vi "MeasLeakRate11.vi"() -> ()   [LabVIEW 2011]
panel:
  out "fit":cluster{"element":dbl, "Value":dbl}[](array[cluster])
  out "T-T0,P":cluster{"element":dbl, "element":dbl}[](array[cluster])
  out "t0":dbl format="%#_8f"
  out "XY Graph":T1(graph)
  out "S00":i32
  out "S20":dbl
  out "S11":dbl
  out "S10":dbl
  out "S01":dbl
  out "T,P":cluster{"element":dbl, "element":dbl}[](array[cluster])
  out "dPdt":dbl
  out "P0":dbl
  out "average P (Torr)":string
  in  "Control Valve local":bool
  in  "Exhaust Local":bool
  in  "Exhaust Close":bool
  in  "Exhaust Open":bool
  in  "Control Close":bool
  in  "Control Open":bool
  in  "reset":bool
  in  "# points to watch":i32=60
  out "leak rate (Torr/min)":string
  out "P":dbl
  out "first":bool=TRUE
  in  "interval (s)":dbl=0.5
  in  "stop":bool
  out "P(Torr)":string
  # "Pressure control valve:"
  # "Exahaust valve:"
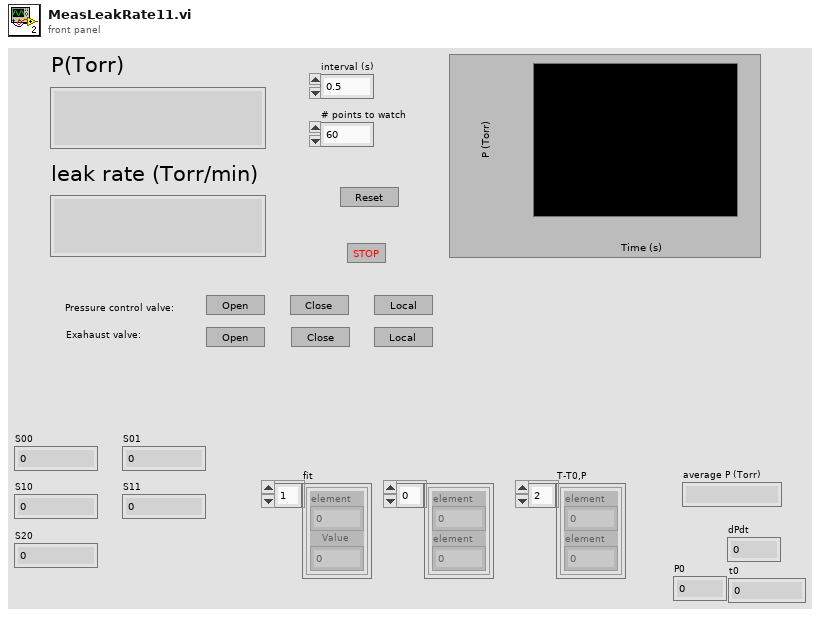
[diagram p1: front panel]
types:
  T1 = cluster{"Value":cluster{"element":dbl, "element":dbl}[]}[]
  T2 = cluster{"Value":cluster{"element":dbl, "Value":dbl}[]}[]
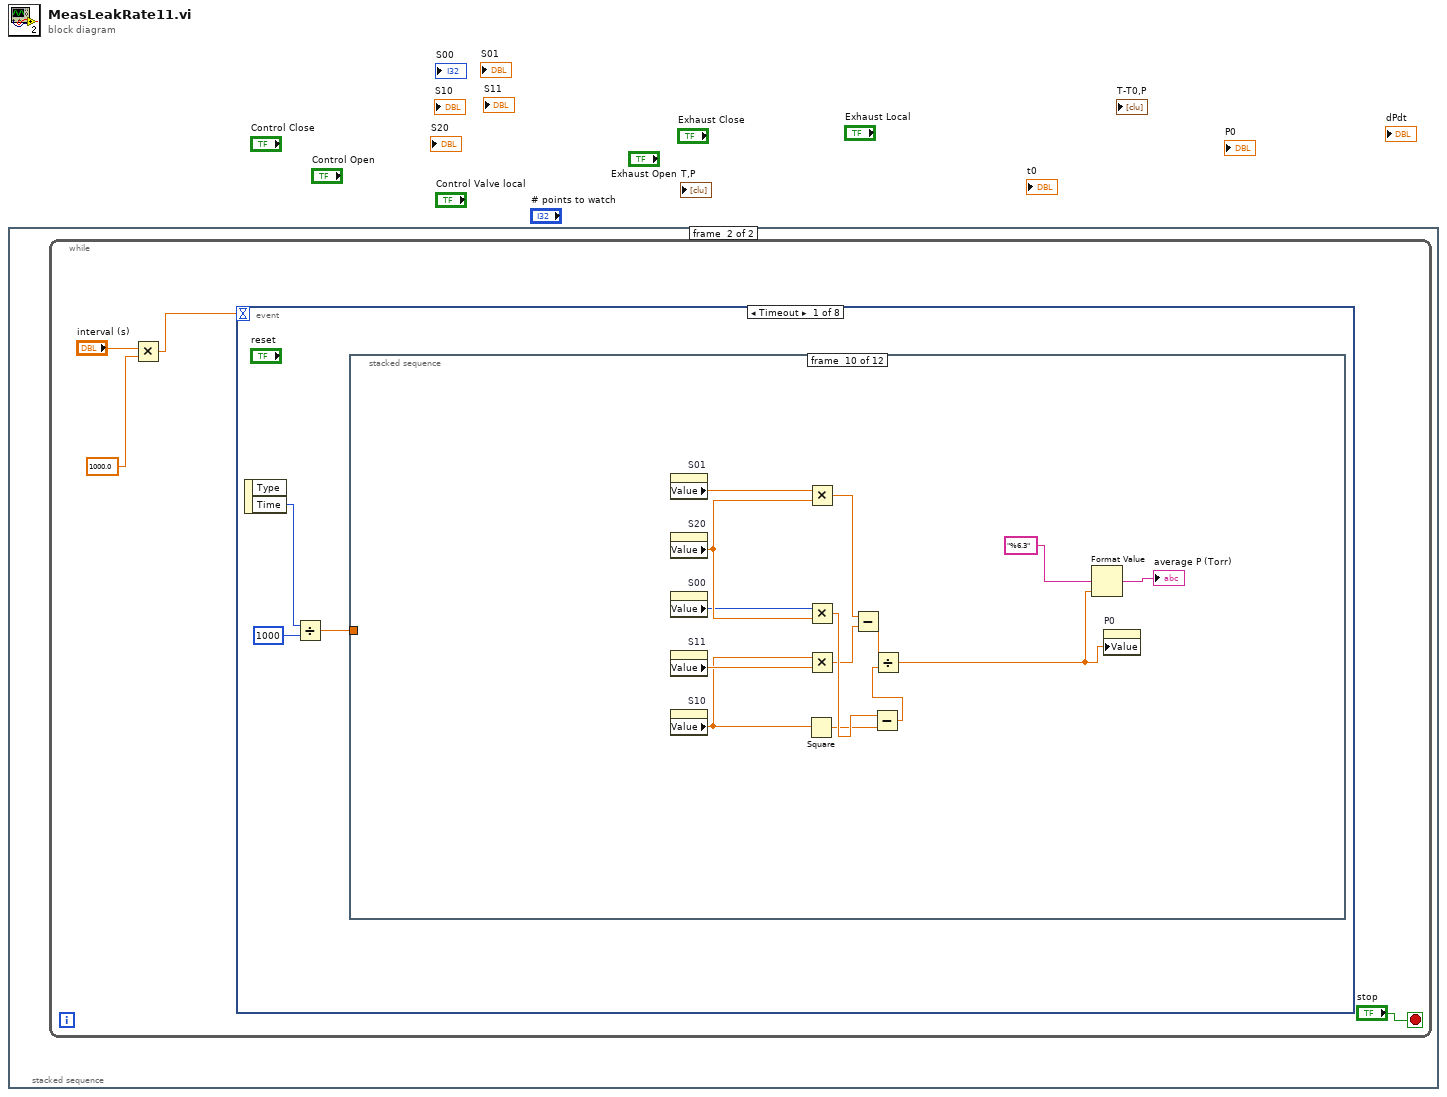
[diagram p0: block diagram]
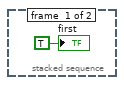
[diagram p2: hidden frame]
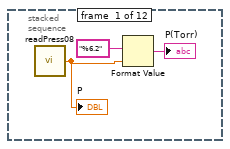
[diagram p3: hidden frame]
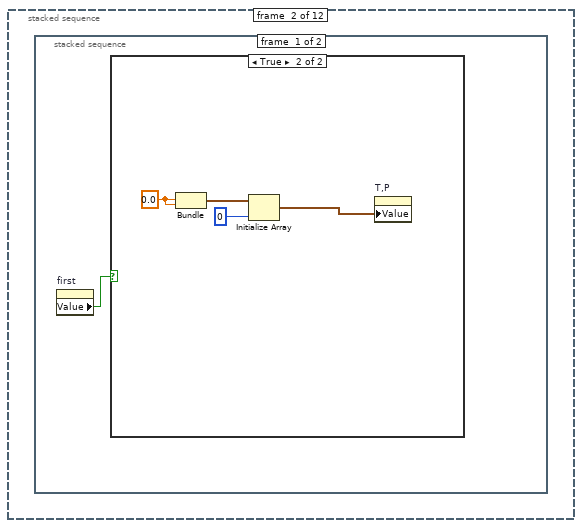
[diagram p4: hidden frame]
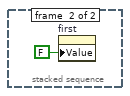
[diagram p6: hidden frame]
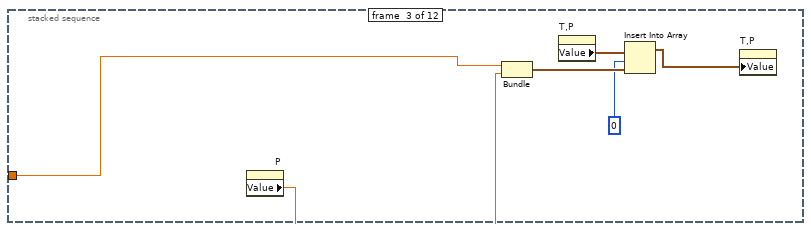
[diagram p7: hidden frame]
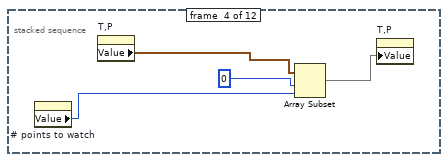
[diagram p8: hidden frame]
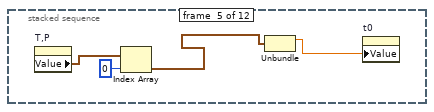
[diagram p9: hidden frame]
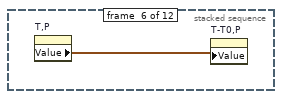
[diagram p10: hidden frame]
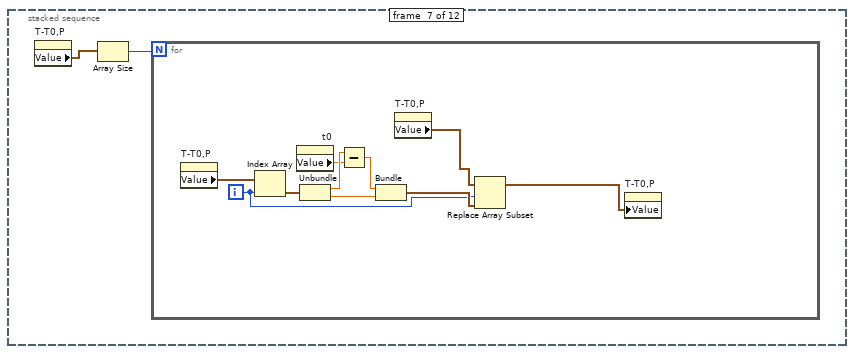
[diagram p11: hidden frame]
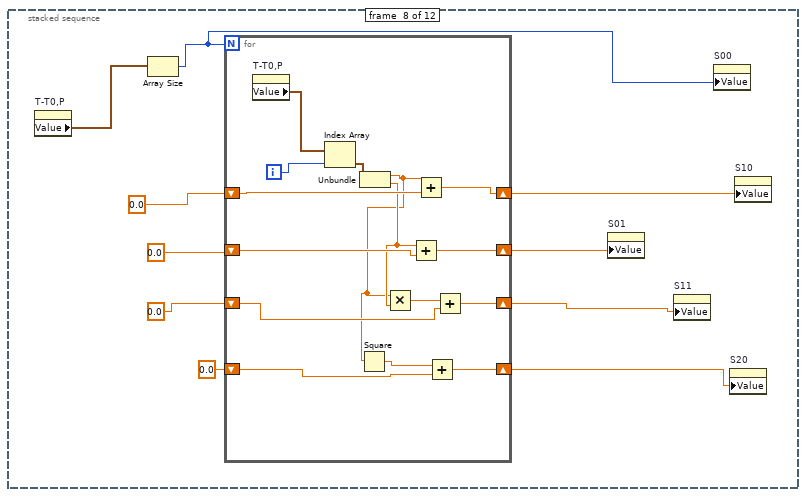
[diagram p12: hidden frame]
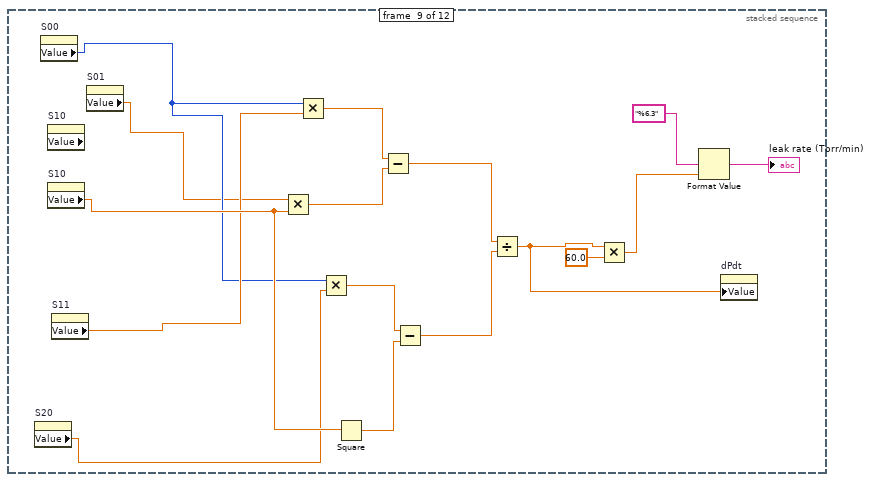
[diagram p13: hidden frame]
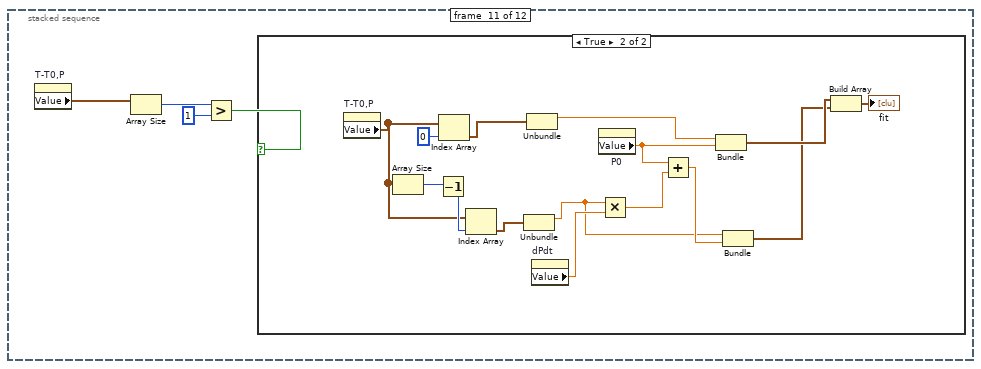
[diagram p14: hidden frame]
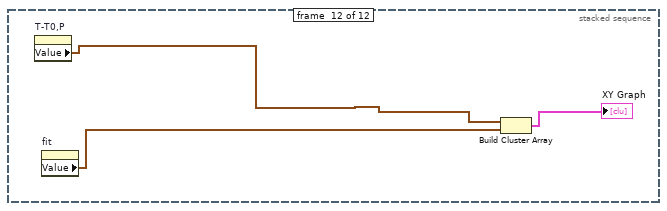
[diagram p16: hidden frame]
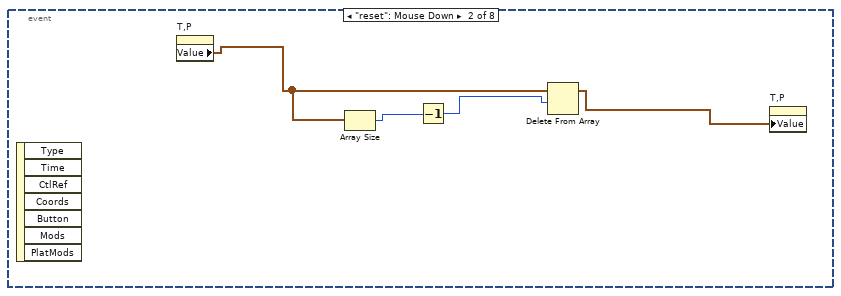
[diagram p17: hidden frame]
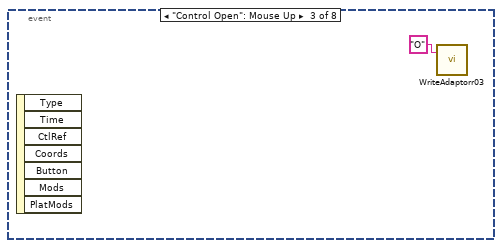
[diagram p18: hidden frame]
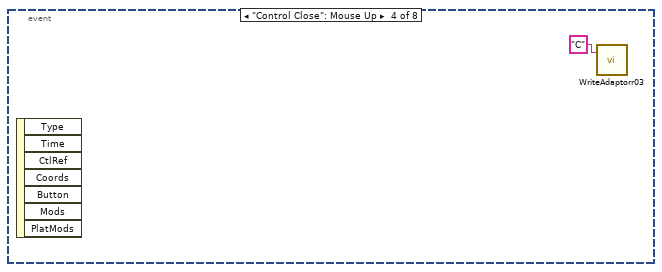
[diagram p19: hidden frame]
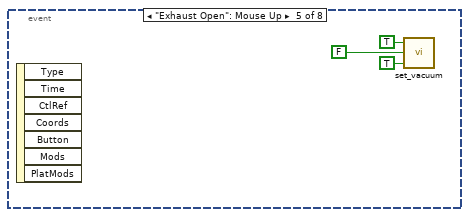
[diagram p20: hidden frame]
diagram:
  n1 = stacked-sequence {
    frame #0 {
      "first" <- TRUE ("first")
    }
    frame #1 {
      n2 = while {
        stop <- "stop" stop-if-true
        n3 = Multiply(x="interval (s)", y=1000.0) -> (x*y=w3:dbl)
        n4 = event shown="[0] Timeout" {
          selector: _ -> [_ _ _ _ _ _ _ _]
          dyn-events: _ -> [_ _ _ _ _ _ _ _]
          timeout: w3 -> [_ _ _ _ _ _ _ _]
          event Timeout {
            n5 = event-data() -> ("Time"=w8:u32)  [unwired: 1 in, 1 out]
            n6 = Divide(x=w8, y=u32 1000) -> (x/y=w6:dbl)
            n7 = stacked-sequence {
              tunnel: w6 -> [_ _ w23 _ _ _ _ _ _ _ _ _]
              frame #0 {
                n8 = call "readPress08.vi"() -> ("P"=w10:dbl)
                "P" <- w10
                n9 = Format Value(format string="%6.2", value (0)=w10) -> (output string=→"P(Torr)":string)  [unwired: 1 in]
              }
              frame #1 {
                n10 = stacked-sequence {
                  frame #0 {
                    n11 = property on="first" class="Bool (strict)"() -> ("Value"=w12:bool)  [unwired: 2 in, 2 out]
                    n12 = case shown="True" w12 {
                      frame False {
                      }
                      frame True {
                        w15 = 0.0 ("element")
                        n13 = Bundle("element"=w15, "element"=w15) -> (w14:cluster{"element":dbl, "element":dbl})  [unwired: 1 in]
                        n14 = Initialize Array(w14, 0 ("dimension size")) -> (w13:cluster{"element":dbl, "element":dbl}[])
                        n15 = property on="T,P" class="Arr (strict)"("Value"=w13) -> ()  [unwired: 2 in, 2 out]
                      }
                    }
                  }
                  frame #1 {
                    n16 = property on="first" class="Bool (strict)"("Value"=FALSE ("first")) -> ()  [unwired: 2 in, 2 out]
                  }
                }
              }
              frame #2 {
                n17 = property on="P" class="DigNum (strict)"() -> ("Value"=w22:dbl)  [unwired: 2 in, 2 out]
                n18 = Bundle(w23, "Value"=w22) -> (w20:cluster{dbl, "Value":dbl})  [unwired: 1 in]
                n19 = property on="T,P" class="Arr (strict)"() -> ("Value"=w21:cluster{"element":dbl, "element":dbl}[])  [unwired: 2 in, 2 out]
                n20 = Insert Into Array(array=w21, index=0, new element=w20) -> (w18:cluster{"element":dbl, "element":dbl}[])
                n21 = property on="T,P" class="Arr (strict)"("Value"=w18) -> ()  [unwired: 2 in, 2 out]
              }
              frame #3 {
                n22 = property on="# points to watch" class="DigNum (strict)"() -> ("Value"=w25:i32)  [unwired: 2 in, 2 out]
                n23 = property on="T,P" class="Arr (strict)"() -> ("Value"=w26:cluster{"element":dbl, "element":dbl}[])  [unwired: 2 in, 2 out]
                n24 = Array Subset(array=w26, index=0, length=w25) -> (w24:cluster{"element":dbl, "element":dbl}[])
                n25 = property on="T,P" class="Arr (strict)"("Value"=w24) -> ()  [unwired: 2 in, 2 out]
              }
              frame #4 {
                n26 = property on="T,P" class="Arr (strict)"() -> ("Value"=w31:cluster{"element":dbl, "element":dbl}[])  [unwired: 2 in, 2 out]
                n27 = Index Array(array=w31, index=0) -> (element=w29:cluster{"element":dbl, "element":dbl})
                n28 = Unbundle(w29) -> ("element"=w28:dbl)  [unwired: 1 out]
                n29 = property on="t0" class="DigNum (strict)"("Value"=w28) -> ()  [unwired: 2 in, 2 out]
              }
              frame #5 {
                n30 = property on="T,P" class="Arr (strict)"() -> ("Value"=w32:cluster{"element":dbl, "element":dbl}[])  [unwired: 2 in, 2 out]
                n31 = property on="T-T0,P" class="Arr (strict)"("Value"=w32) -> ()  [unwired: 2 in, 2 out]
              }
              frame #6 {
                n32 = property on="T-T0,P" class="Arr (strict)"() -> ("Value"=w34:cluster{"element":dbl, "element":dbl}[])  [unwired: 2 in, 2 out]
                n33 = Array Size(array=w34) -> (size(s)=w33:i32)
                n34 = for {
                  N: w33 -> [_]
                  i -> [w35]
                  n35 = property on="T-T0,P" class="Arr (strict)"() -> ("Value"=w39:cluster{"element":dbl, "element":dbl}[])  [unwired: 2 in, 2 out]
                  n36 = Index Array(array=w39, index=w35) -> (element=w44:cluster{"element":dbl, "element":dbl})
                  n37 = property on="t0" class="DigNum (strict)"() -> ("Value"=w42:dbl)  [unwired: 2 in, 2 out]
                  n38 = Unbundle(w44) -> ("element"=w43:dbl, "element"=w40:dbl)
                  n39 = Subtract(x=w43, y=w42) -> (x-y=w41:dbl)
                  n40 = Bundle(w41, "element"=w40) -> (w38:cluster{dbl, "element":dbl})  [unwired: 1 in]
                  n41 = property on="T-T0,P" class="Arr (strict)"() -> ("Value"=w37:cluster{"element":dbl, "element":dbl}[])  [unwired: 2 in, 2 out]
                  n42 = Replace Array Subset(array=w37, new element=w38, index=w35) -> (w36:cluster{"element":dbl, "element":dbl}[])
                  n43 = property on="T-T0,P" class="Arr (strict)"("Value"=w36) -> ()  [unwired: 2 in, 2 out]
                }
              }
              frame #7 {
                n44 = property on="T-T0,P" class="Arr (strict)"() -> ("Value"=w45:cluster{"element":dbl, "element":dbl}[])  [unwired: 2 in, 2 out]
                n45 = Array Size(array=w45) -> (size(s)=w49:i32)
                n46 = for {
                  N: w49 -> [_]
                  shift-right: [w67] -> w48
                  shift-left: 0.0 -> [w69]
                  shift-right: [w66] -> w52
                  shift-left: 0.0 -> [w65]
                  shift-right: [w62] -> w47
                  shift-left: 0.0 -> [w61]
                  shift-right: [w58] -> w46
                  shift-left: 0.0 -> [w57]
                  i -> [w56]
                  n47 = property on="T-T0,P" class="Arr (strict)"() -> ("Value"=w55:cluster{"element":dbl, "element":dbl}[])  [unwired: 2 in, 2 out]
                  n48 = Index Array(array=w55, index=w56) -> (element=w68:cluster{"element":dbl, "element":dbl})
                  n49 = Unbundle(w68) -> ("element"=w60:dbl, "element"=w64:dbl)
                  n50 = Square(x=w60) -> (x^2=w59:dbl)
                  n51 = Multiply(x=w60, y=w64) -> (x*y=w63:dbl)
                  n52 = Add(x=w64, y=w65) -> (x+y=w66:dbl)
                  n53 = Add(x=w60, y=w69) -> (x+y=w67:dbl)
                  n54 = Add(x=w59, y=w57) -> (x+y=w58:dbl)
                  n55 = Add(x=w63, y=w61) -> (x+y=w62:dbl)
                }
                n56 = property on="S01" class="DigNum (strict)"("Value"=w52) -> ()  [unwired: 2 in, 2 out]
                n57 = property on="S11" class="DigNum (strict)"("Value"=w47) -> ()  [unwired: 2 in, 2 out]
                n58 = property on="S00" class="DigNum (strict)"("Value"=w49) -> ()  [unwired: 2 in, 2 out]
                n59 = property on="S20" class="DigNum (strict)"("Value"=w46) -> ()  [unwired: 2 in, 2 out]
                n60 = property on="S10" class="DigNum (strict)"("Value"=w48) -> ()  [unwired: 2 in, 2 out]
              }
              frame #8 {
                n61 = property on="S20" class="DigNum (strict)"() -> ("Value"=w73:dbl)  [unwired: 2 in, 2 out]
                n62 = property on="S00" class="DigNum (strict)"() -> ("Value"=w72:i32)  [unwired: 2 in, 2 out]
                n63 = property on="S10" class="DigNum (strict)" props=["Value"]() -> ()  [unwired: 2 in, 3 out]
                n64 = property on="S10" class="DigNum (strict)"() -> ("Value"=w75:dbl)  [unwired: 2 in, 2 out]
                n65 = property on="S11" class="DigNum (strict)"() -> ("Value"=w74:dbl)  [unwired: 2 in, 2 out]
                n66 = property on="S01" class="DigNum (strict)"() -> ("Value"=w71:dbl)  [unwired: 2 in, 2 out]
                n67 = Multiply(x=w71, y=w75) -> (x*y=w84:dbl)
                n68 = Multiply(x=w72, y=w74) -> (x*y=w85:dbl)
                n69 = Multiply(x=w72, y=w73) -> (x*y=w83:dbl)
                n70 = Square(x=w75) -> (x^2=w82:dbl)
                n71 = Subtract(x=w85, y=w84) -> (x-y=w81:dbl)
                n72 = Subtract(x=w83, y=w82) -> (x-y=w80:dbl)
                n73 = Divide(x=w81, y=w80) -> (x/y=w70:dbl)
                n74 = Multiply(x=w70, y=60.0) -> (x*y=w76:dbl)
                n75 = Format Value(format string="%6.3", value (0)=w76) -> (output string=→"leak rate (Torr/min)":string)  [unwired: 1 in]
                n76 = property on="dPdt" class="DigNum (strict)"("Value"=w70) -> ()  [unwired: 2 in, 2 out]
              }
              frame #9 {
                n77 = property on="S01" class="DigNum (strict)"() -> ("Value"=w99:dbl)  [unwired: 2 in, 2 out]
                n78 = property on="S20" class="DigNum (strict)"() -> ("Value"=w96:dbl)  [unwired: 2 in, 2 out]
                n79 = property on="S00" class="DigNum (strict)"() -> ("Value"=w95:i32)  [unwired: 2 in, 2 out]
                n80 = property on="S11" class="DigNum (strict)"() -> ("Value"=w98:dbl)  [unwired: 2 in, 2 out]
                n81 = property on="S10" class="DigNum (strict)"() -> ("Value"=w97:dbl)  [unwired: 2 in, 2 out]
                n82 = Square(x=w97) -> (x^2=w89:dbl)
                n83 = Multiply(x=w99, y=w96) -> (x*y=w87:dbl)
                n84 = Multiply(x=w95, y=w96) -> (x*y=w90:dbl)
                n85 = Multiply(x=w97, y=w98) -> (x*y=w86:dbl)
                n86 = Subtract(x=w87, y=w86) -> (x-y=w94:dbl)
                n87 = Subtract(x=w90, y=w89) -> (x-y=w88:dbl)
                n88 = Divide(x=w94, y=w88) -> (x/y=w91:dbl)
                n89 = Format Value(format string="%6.3", value (0)=w91) -> (output string=→"average P (Torr)":string)  [unwired: 1 in]
                n90 = property on="P0" class="DigNum (strict)"("Value"=w91) -> ()  [unwired: 2 in, 2 out]
              }
              frame #10 {
                n91 = property on="T-T0,P" class="Arr (strict)"() -> ("Value"=w103:cluster{"element":dbl, "element":dbl}[])  [unwired: 2 in, 2 out]
                n92 = Array Size(array=w103) -> (size(s)=w102:i32)
                n93 = Greater?(x=w102, y=1) -> (0:w100:bool)
                n94 = case shown="True" w100 {
                  frame False {
                  }
                  frame True {
                    n95 = property on="T-T0,P" class="Arr (strict)"() -> ("Value"=w107:cluster{"element":dbl, "element":dbl}[])  [unwired: 2 in, 2 out]
                    n96 = Array Size(array=w107) -> (size(s)=w117:i32)
                    n97 = Decrement(x=w117) -> (x-1=w116:i32)
                    n98 = Index Array(array=w107, index=0) -> (element=w115:cluster{"element":dbl, "element":dbl})
                    n99 = Index Array(array=w107, index=w116) -> (element=w114:cluster{"element":dbl, "element":dbl})
                    n100 = Unbundle(w114) -> ("element"=w108:dbl)  [unwired: 1 out]
                    n101 = Unbundle(w115) -> ("element"=w110:dbl)  [unwired: 1 out]
                    n102 = property on="dPdt" class="DigNum (strict)"() -> ("Value"=w113:dbl)  [unwired: 2 in, 2 out]
                    n103 = property on="P0" class="DigNum (strict)"() -> ("Value"=w111:dbl)  [unwired: 2 in, 2 out]
                    n104 = Multiply(x=w108, y=w113) -> (x*y=w112:dbl)
                    n105 = Add(x=w111, y=w112) -> (x+y=w109:dbl)
                    n106 = Bundle("element"=w110, "Value"=w111) -> (w106:cluster{"element":dbl, "Value":dbl})  [unwired: 1 in]
                    n107 = Bundle("element"=w108, w109) -> (w105:cluster{"element":dbl, dbl})  [unwired: 1 in]
                    n108 = Build Array(w106, w105) -> (→"fit":cluster{"element":dbl, "Value":dbl}[])
                  }
                }
              }
              frame #11 {
                n109 = property on="T-T0,P" class="Arr (strict)"() -> ("Value"=w121:cluster{"element":dbl, "element":dbl}[])  [unwired: 2 in, 2 out]
                n110 = property on="fit" class="Arr (strict)"() -> ("Value"=w119:cluster{"element":dbl, "Value":dbl}[])  [unwired: 2 in, 2 out]
                n111 = Build Cluster Array(w121, w119) -> (→"XY Graph":T2)
              }
            }
          }
          event "reset": Mouse Down {
            n112 = event-data() -> ()  [unwired: 1 in, 7 out]
            n113 = property on="T,P" class="Arr (strict)"() -> ("Value"=w123:cluster{"element":dbl, "element":dbl}[])  [unwired: 2 in, 2 out]
            n114 = Array Size(array=w123) -> (size(s)=w125:i32)
            n115 = Decrement(x=w125) -> (x-1=w124:i32)
            n116 = Delete From Array(array=w123, length=w124) -> (array with subset deleted=w122:cluster{"element":dbl, "element":dbl}[])  [unwired: 1 in, 1 out]
            n117 = property on="T,P" class="Arr (strict)"("Value"=w122) -> ()  [unwired: 2 in, 2 out]
          }
          event "Control Open": Mouse Up {
            n118 = event-data() -> ()  [unwired: 1 in, 7 out]
            n119 = call "WriteAdaptorr03.vi"("string to write"="O") -> ()  [unwired: 1 in, 1 out]
          }
          event "Control Close": Mouse Up {
            n120 = event-data() -> ()  [unwired: 1 in, 7 out]
            n121 = call "WriteAdaptorr03.vi"("string to write"="C") -> ()  [unwired: 1 in, 1 out]
          }
          event "Exhaust Open": Mouse Up {
            n122 = event-data() -> ()  [unwired: 1 in, 7 out]
            n123 = call "set_vacuum.vi"("Vac Remote"=TRUE, "Atm Exhaust"=FALSE, "Vac Exhaust"=TRUE) -> ()
          }
          event "Exhaust Close": Mouse Up {
            n124 = event-data() -> ()  [unwired: 1 in, 7 out]
            n125 = call "set_vacuum.vi"("Vac Remote"=TRUE, "Atm Exhaust"=FALSE, "Vac Exhaust"=FALSE) -> ()
          }
          event "Exhaust Local": Mouse Up {
            n126 = event-data() -> ()  [unwired: 1 in, 7 out]
            n127 = call "set_vacuum.vi"() -> ()  [unwired: 3 in]
          }
          event "Control Valve local": Mouse Down? {
            n128 = event-data() -> ()  [unwired: 1 in, 7 out]
            n129 = call "WriteAdaptorr03.vi"("string to write"="D5") -> ()  [unwired: 1 in, 1 out]
            n130 = event-data() -> ()  [unwired: 5 in, 1 out]
          }
        }
      }
    }
  }
